vi "Is AO Timing Parameter Changed.vi"(8 "error in (no error)":errorcluster, 11 "Generator in":refnum<class "Generator.lvclass">) -> (0 "error out":errorcluster, 2 "AO frequency or phase or function changed?":bool, 3 "Generator out":refnum<class "Generator.lvclass">)   [LabVIEW 2019, in "Generator.lvclass"]
uses:
  Generator.lvclass
  Generator.lvclass/Generator.ctl
  2d279565-7099-49c8-81b4-f6f9d5ffada6.vi
  0a297234-f1a7-4d57-8c2f-a53db9f138df.vi
  5b7423eb-c88a-4eec-af7d-cb9347c02f62.vi
  e3b7d657-e47f-4a13-bbc2-a12aee264466.vi
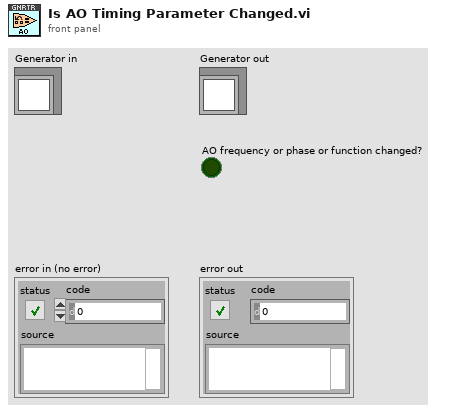
[diagram p1: front panel]
types:
  T1 = typedef "Generator.lvclass/AO.Channel--Cluster--Array.ctl" = T2[]
  T2 = typedef "Generator.lvclass/AO.Channel--Cluster.ctl" = cluster{"Enable?":bool, "Channel":i32, "Amplitude":dbl, "Offset":dbl, "Frequency":dbl, "Phase":dbl, "Function":T3, "Sweeping?":bool, "Limit AC?":bool, "Limit DC?":bool, "Duty Cycle?":bool, "Duty Cycle":dbl}
  T3 = typedef "Generator.lvclass/AO.Channel.Function--Enum.ctl" = enum16{"sine", "square", "triangle", "saw"}
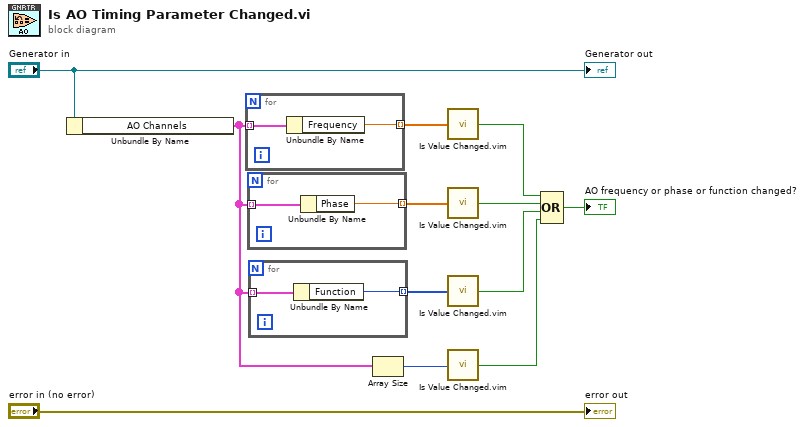
[diagram p0: block diagram]
diagram:
  n1 = Unbundle By Name("Generator in") -> ("AO Channels"=w8:T1)
  n2 = for {
    tunnel: w8 -> [w14] mode=indexing
    tunnel: [w13] -> w2 mode=indexing
    n3 = Unbundle By Name(w14) -> ("Frequency"=w13:dbl)
  }
  n4 = for {
    tunnel: w8 -> [w16] mode=indexing
    tunnel: [w15] -> w6 mode=indexing
    n5 = Unbundle By Name(w16) -> ("Phase"=w15:dbl)
  }
  n6 = for {
    tunnel: w8 -> [w18] mode=indexing
    tunnel: [w17] -> w5 mode=indexing
    n7 = Unbundle By Name(w18) -> ("Function"=w17:T3)
  }
  n8 = Array Size(array=w8) -> (size(s)=w9:i32)
  n9 = call "Is Value Changed.vim"("value"=w2) -> ("changed or first call?"=w1:bool)
  n10 = call "Is Value Changed.vim"("value"=w6) -> ("changed or first call?"=w3:bool)
  n11 = call "Is Value Changed.vim"("value"=w5) -> ("changed or first call?"=w4:bool)
  n12 = call "Is Value Changed.vim"("value"=w9) -> ("changed or first call?"=w7:bool)
  n13 = Compound Arithmetic op=OR(w1, w3, w4, w7) -> (→"AO frequency or phase or function changed?":bool)
  "error out" <- "error in (no error)"
  "Generator out" <- "Generator in"
